vi "Vertical_Spread_string.vi"(1 "Index":i32, 2 "Sigma name":string) -> (0 "resulting string":string)   [LabVIEW 2011]
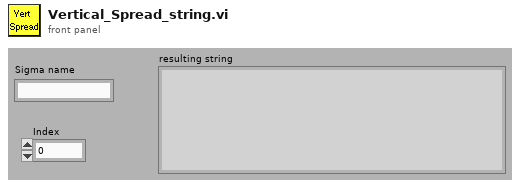
[diagram p1: front panel]
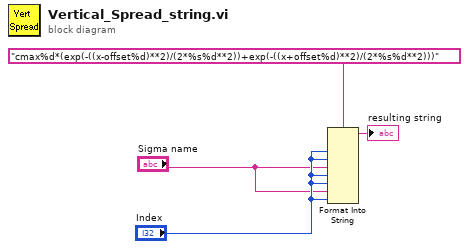
[diagram p0: block diagram]
diagram:
  n1 = Format Into String(format string="cmax%d*(exp(-((x-offset%d)**2)/(2*%s%d**2))+exp(-((x+offset%d)**2)/(2*%s%d**2)))", "Index", "Index", "Sigma name", "Index", "Index", "Sigma name", "Index") -> (resulting string=→"resulting string":string)  [unwired: 2 in, 1 out]
